vi "Configure magnetometer.vi"(8 "error in (no error)":errorcluster, 11 "Accelerometer":T1) -> (0 "error out":errorcluster, 3 "Accelerometer out":T1, 4 "whoami":u8 format="%.0b")   [LabVIEW 2013]
doc: "Use this template to build a VI to use as a subVI."
uses:
  AccelerometerSPI.ctl
  <vilib>/ni845x/ni845x.llb/ni845xControl.ctl
  <vilib>/ni845x/ni845x.llb/ni845xSpiConfiguration.ctl
panel:
  out "read data 0":u8[](array[numeric]) format="%.0b"
  out "read data 2":u8[](array[numeric]) format="%.0b"
  out "read data 1":u8[](array[numeric]) format="%.0x"
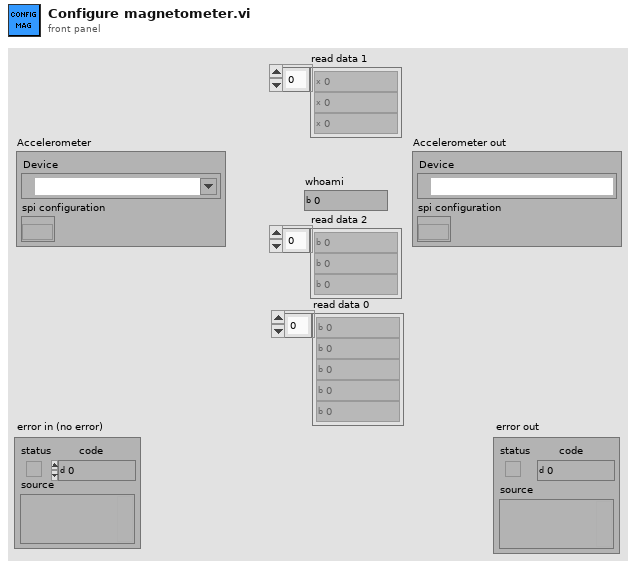
[diagram p1: front panel]
types:
  T1 = typedef "AccelerometerSPI.ctl" = cluster{"Device":T2, "spi configuration":T3}
  T2 = typedef "ni845xControl.ctl" = refnum<k21>
  T3 = typedef "ni845xSpiConfiguration.ctl" = refnum<k20>
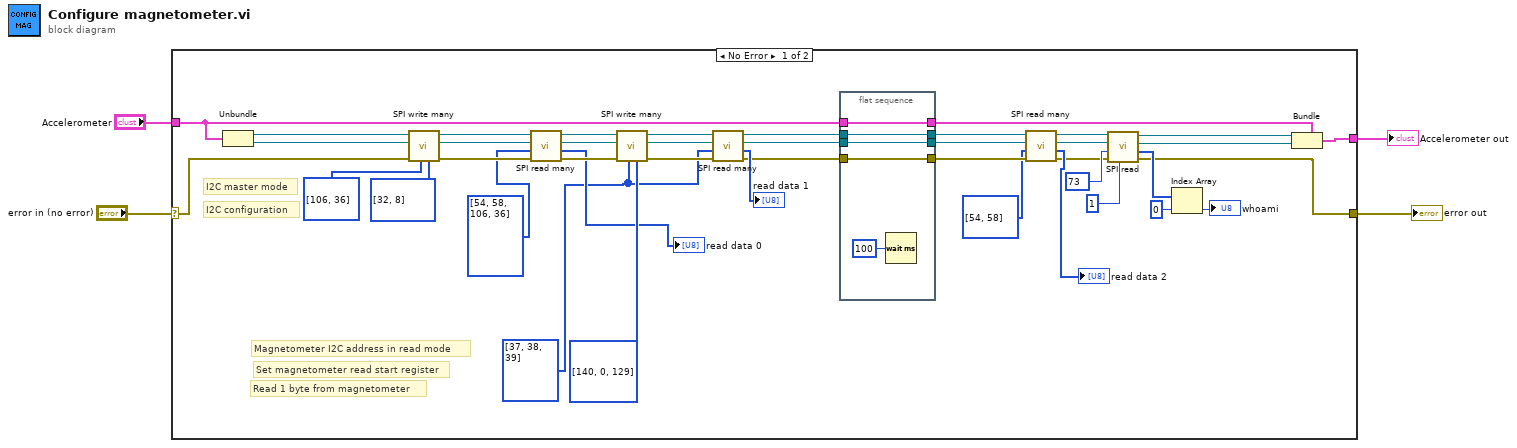
[diagram p0: block diagram]
diagram:
  n1 = case shown="No Error" "error in (no error)" {
    selector: "error in (no error)" -> [w41 w52]
    tunnel: [w34 w52] -> w3
    tunnel: "Accelerometer" -> [w26 w51]
    tunnel: [w45 w51] -> w1
    frame No Error {
      w5 = u8[] [37, 38, 39] ("addresses")
      # "Read 1 byte from magnetometer"
      # "Set magnetometer read start register"
      # "Magnetometer I2C address in read mode"
      # "I2C configuration"
      # "I2C master mode"
      n2 = Unbundle(w26) -> ("Device"=w43:T2, "spi configuration"=w42:T3)
      n3 = call "SPI write many.vi"("values"=u8[] [32, 8] ("addresses"), "addresses"=u8[] [106, 36], "error in (no error)"=w41, "spi configuration in"=w42, "Device ref in"=w43) -> ("error out"=w11:errorcluster, "spi configuration out"=w12:T3, "Device ref out"=w13:T2)  [unwired: 4 in]
      n4 = call "SPI read many.vi"("error in (no error)"=w11, "Addresses"=u8[] [54, 58, 106, 36] ("addresses"), "spi configuration in"=w12, "Device ref in"=w13) -> ("error out"=w8:errorcluster, "read data"=→"read data 0":u8[], "spi configuration out"=w9:T3, "Device ref out"=w10:T2)  [unwired: 4 in]
      n5 = call "SPI write many.vi"("values"=u8[] [140, 0, 129] ("addresses"), "addresses"=w5, "error in (no error)"=w8, "spi configuration in"=w9, "Device ref in"=w10) -> ("error out"=w27:errorcluster, "spi configuration out"=w29:T3, "Device ref out"=w30:T2)  [unwired: 4 in]
      n6 = call "SPI read many.vi"("error in (no error)"=w27, "Addresses"=w5, "spi configuration in"=w29, "Device ref in"=w30) -> ("error out"=w23:errorcluster, "read data"=→"read data 1":u8[], "spi configuration out"=w24:T3, "Device ref out"=w25:T2)  [unwired: 4 in]
      n7 = flat-sequence {
        tunnel: w26 -> [w49]
        tunnel: w25 -> [w48]
        tunnel: w24 -> [w47]
        tunnel: w23 -> [w46]
        tunnel: [w49] -> w22
        tunnel: [w48] -> w21
        tunnel: [w47] -> w20
        tunnel: [w46] -> w19
        frame #0 {
          n8 = Wait (ms)(milliseconds to wait=u32 100) -> ()  [unwired: 1 out]
        }
      }
      n9 = call "SPI read many.vi"("error in (no error)"=w19, "Addresses"=u8[] [54, 58] ("addresses"), "spi configuration in"=w20, "Device ref in"=w21) -> ("error out"=w16:errorcluster, "read data"=→"read data 2":u8[], "spi configuration out"=w15:T3, "Device ref out"=w14:T2)  [unwired: 4 in]
      n10 = call "SPI read.vi"("Number of bytes"=1, "error in (no error)"=w16, "Address"=u8 73, "spi configuration in"=w15, "Device ref in"=w14) -> ("error out"=w34:errorcluster, "read data"=w37:u8[], "spi configuration out"=w33:T3, "Device ref out"=w32:T2)  [unwired: 3 in]
      n11 = Index Array(array=w37, index=0) -> (element=→"whoami":u8)
      n12 = Bundle(cluster=w22, "Device"=w32, "spi configuration"=w33) -> (w45:T1)
    }
    frame Error {
    }
  }
  "error out" <- w3
  "Accelerometer out" <- w1
